vi "SenderCaller.vi"() -> ()   [LabVIEW 2014]
uses:
  CommMsg.ctl
panel:
  in  "stop":bool
  in  "Slide":dbl(slide) scale=0.0..10.0
  in  "IP Address":string="localhost"
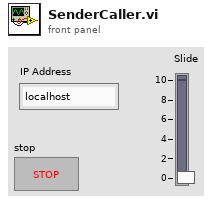
[diagram p1: front panel]
types:
  T1 = typedef "CommMsg.ctl" = cluster{"cmd":enum16{"exit", "data"}, "value":variant}
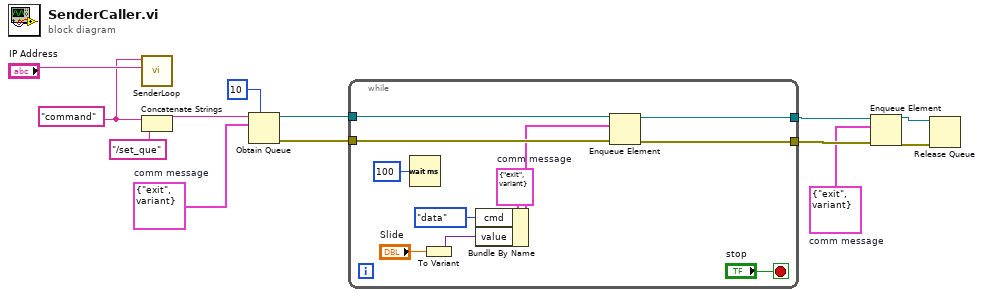
[diagram p0: block diagram]
diagram:
  w3 = T1 {"cmd"=enum."exit", "value"=variant}  # comm message
  w8 = T1 {"cmd"=enum."exit", "value"=variant}  # comm message
  w11 = "command" ("name")
  n1 = call "SenderLoop.vi"("IP Address"="IP Address", "name"=w11) -> ()  [unwired: 10 in]
  n2 = Concatenate Strings(w11, "/set_que" ("writer name")) -> (w9:string)
  n3 = Obtain Queue(max queue size (-1, unlimited)=10, name (unnamed)=w9, element data type=w8) -> (queue out=w7:refnum<queue>, error out=w6:errorcluster)  [unwired: 2 in, 1 out]
  n4 = while {
    tunnel: w7 -> [w24]
    tunnel: w6 -> [w23]
    tunnel: [w15] -> w5
    tunnel: [w14] -> w4
    stop <- "stop" stop-if-true
    w21 = T1 {"cmd"=enum."exit", "value"=variant}  # comm message
    n5 = Wait (ms)(milliseconds to wait=u32 100) -> ()  [unwired: 1 out]
    n6 = To Variant(anything="Slide") -> (Variant=w20:variant)
    n7 = Bundle By Name(cluster=w21, "cmd"=enum16{"exit", "data"}."data", "value"=w20) -> (w18:T1)
    n8 = Enqueue Element(queue=w24, element=w18, error in (no error)=w23) -> (queue out=w15:refnum<queue>, error out=w14:errorcluster)  [unwired: 1 in, 1 out]
  }
  n9 = Enqueue Element(queue=w5, element=w3, error in (no error)=w4) -> (queue out=w2:refnum<queue>, error out=w1:errorcluster)  [unwired: 1 in, 1 out]
  n10 = Release Queue(queue=w2, error in (no error)=w1) -> ()  [unwired: 1 in, 3 out]
